vi "Append New Sheet.vi"(6 "Set as active (T)":bool=TRUE, 8 "error in (no error)":errorcluster, 10 "Sheet Name":string, 11 "MS-Excel in":refnum<class "MS-Excel.lvclass">) -> (0 "error out":errorcluster, 1 "Created?":bool, 2 "Created Sheet Name":string, 3 "MS-Excel out":refnum<class "MS-Excel.lvclass">)   [LabVIEW 2017, in "LabVIEW NPOI.lvlib" / "MS-Excel.lvclass"]
doc: "Create new sheet to the associated workbook to the <b>Document</b>, nammed <b>SheetName</b>.\n\nNote: \n<b>SheetName</b> is validated to conform to the sheet name rules. If you do not wire this input, the VI generates a automatic worksheet name. \n<b>Set as active</b>: by default the newly created worksheet is becoming the new active worksheet. This behavior will apply even if no worksheet has been created due to the <B>Sheet Name</B> already exists."
uses:
  MS-Excel.lvclass
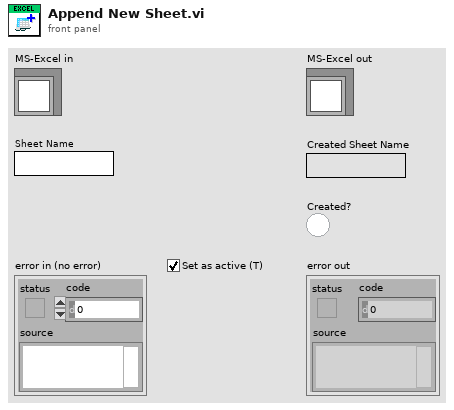
[diagram p1: front panel]
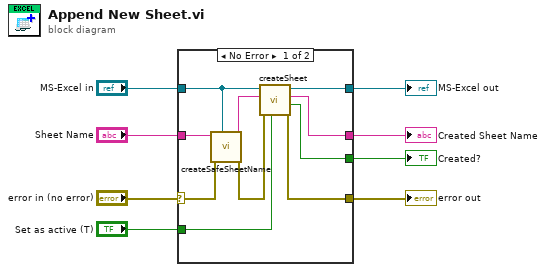
[diagram p0: block diagram]
diagram:
  n1 = case shown="No Error" "error in (no error)" {
    selector: "error in (no error)" -> [w13 w20]
    tunnel: [w17 w20] -> w7
    tunnel: [w18 w19] -> w5
    tunnel: "MS-Excel in" -> [w10 w19]
    tunnel: "Sheet Name" -> [w15 _]
    tunnel: [w16 _] -> w1
    tunnel: "Set as active (T)" -> [w11 _]
    tunnel: [w9 _] -> w2
    frame No Error {
      n2 = call "createSafeSheetName.vi"("MS-Excel in"=w10, "error in (no error)"=w13, "nameProposal"=w15) -> ("error out"=w12:errorcluster, "SafeSheetName"=w14:string)  [unwired: 7 in]
      n3 = call-dynamic "createSheet.vi"("Set as active (T)"=w11, "error in (no error)"=w12, "SheetName"=w14, "MS-Excel in"=w10) -> ("error out"=w17:errorcluster, "Created?"=w9:bool, "Created Sheet Name"=w16:string, "MS-Excel out"=w18:refnum<class "MS-Excel.lvclass">)  [unwired: 4 in]
    }
    frame Error {
    }
  }
  "error out" <- w7
  "MS-Excel out" <- w5
  "Created?" <- w2
  "Created Sheet Name" <- w1
